vi "Dialog_Cannot Edit preset element_Popup.vi"(8 "error in (no error)":errorcluster) -> (0 "error out":errorcluster)   [LabVIEW 2012]
doc: "SciScan 1.2 160622"
panel:
  in  "OK Button":bool
  # "Cannot Edit individual preset elements!\n\n(Note: You need to Edit the top-level Preset command)"
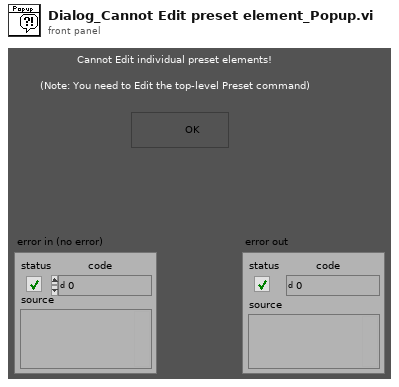
[diagram p1: front panel]
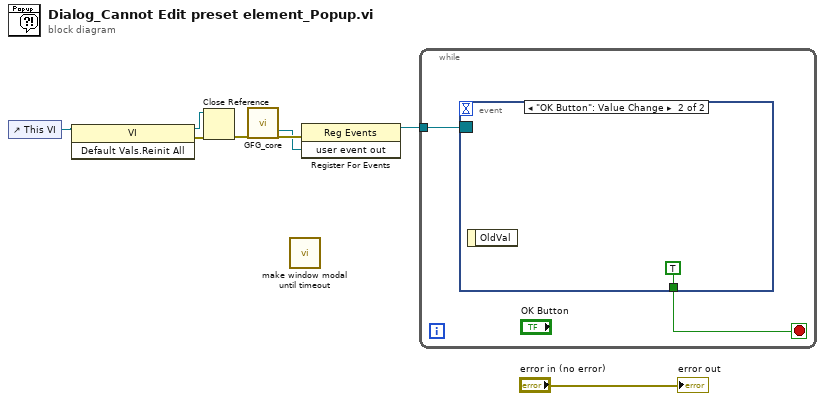
[diagram p0: block diagram]
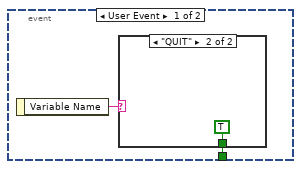
[diagram p2: hidden frame]
diagram:
  n1 = control-ref of="This VI"() -> (w3:refnum<vi>)
  n2 = invoke class="VI" method="Default Vals.Reinit All"(reference=w3) -> (reference out=w1:refnum<vi>, error out=w2:errorcluster)  [unwired: 2 in, 1 out]
  n3 = Close Reference(reference=w1, error in (no error)=w2) -> (error out=w4:errorcluster)
  n4 = call "GFG_core.vi"("error in (no error)"=w4) -> ("user event out"=w7:refnum<user-event>, "error out"=w8:errorcluster)  [unwired: 12 in, 5 out]
  n5 = call "make window modal until timeout.vi"() -> ()  [unwired: 12 in]
  n6 = register-events(error in=w8, w7) -> (reference out=w6:refnum<event-registration>)  [unwired: 1 in, 1 out]
  n7 = while {
    tunnel: w6 -> [w10]
    stop <- w9 stop-if-true
    n8 = event shown="[1] \"OK Button\": Value Change" {
      selector: w10 -> [_ _]
      dyn-events: _ -> [_ _]
      timeout: _ -> [_ _]
      tunnel: [w11 TRUE] -> w9
      event User Event {
        n9 = event-data() -> ("Variable Name"=w12:string)  [unwired: 1 in]
        n10 = case shown="\"QUIT\"" w12 {
          tunnel: [_ TRUE] -> w11
          frame Default {
          }
          frame "QUIT" {
          }
        }
      }
      event "OK Button": Value Change {
        n11 = event-data() -> ()  [unwired: 1 in, 1 out]
      }
    }
  }
  "error out" <- "error in (no error)"
